vi "Passing Paramters 2D Array Of Integers.vi"(9 "cols":i32, 10 "rows":i32, 11 "x":i32) -> (2 "function return":i32, 3 "x out":i32)   [LabVIEW 2018, in "ParsingDataSampleDLL.lvlib"]
doc: "__declspec(dllexport) int PassingParamters_2DArrayOfIntegers (int *x, int rows, int cols);"
uses:
  ParsingDataSampleDLL.lvlib
  ni_reference_vs/Debug/ParsingDataSampleDLL.dll
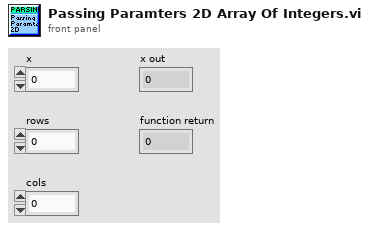
[diagram p1: front panel]
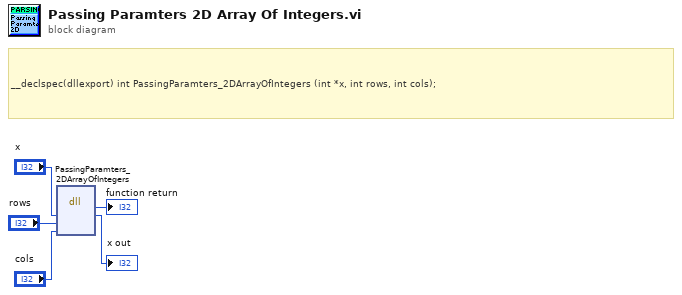
[diagram p0: block diagram]
diagram:
  # "__declspec(dllexport) int PassingParamters_2DArrayOfIntegers (int *x, int rows, int cols);"
  n1 = dll-call lib="C:/Users/celit/Documents/GitHub/Labview_Python_DLL_Call/ni_reference_vs/Debug/ParsingDataSampleDLL.*" fn="PassingParamters_2DArrayOfIntegers"("x"="x", "rows"="rows", "cols"="cols") -> (→"function return":i32, "x"=→"x out":i32)  [unwired: 5 in, 2 out]
